vi "Agilent VNA Read Number of Ports.vi"(7 "Agilent VNA":T1, 8 "error in (no error)":errorcluster, 11 "VISA Resource Name":refnum<visa-resource-name>) -> (0 "error out":errorcluster, 2 "Number of Ports":i8, 3 "dup VISA Resource Name":refnum<visa-resource-name>)   [LabVIEW 2011]
doc: "This VI for the HP 8753 is used to read the sweep type.\n\n0 LINEAR FREQ\n1 LOG FREQ\n2 LIST FREQ\n3 CW TIME\n4 POWER SWEEP"
uses:
  TypeDefs/Agilent VNA Instrument Info.ctl
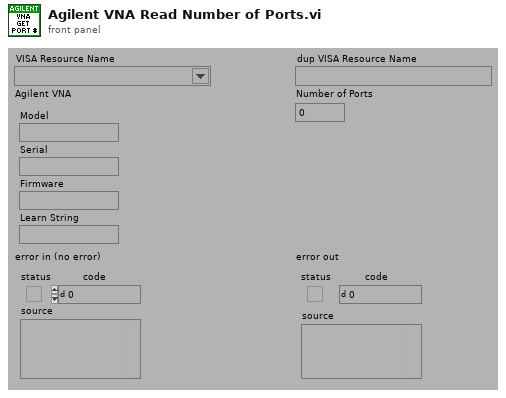
[diagram p1: front panel]
types:
  T1 = typedef "Agilent VNA Instrument Info.ctl" = cluster{"Model":string, "Serial":string, "Firmware":string, "Learn String":string}
  T2 = typedef "Agilent VNA Model.ctl" = enum16{"Not Supported", "8510X", "8719X", "8720X", "8722X", "8753X", "ENA", "PNA", "Field Fox"}
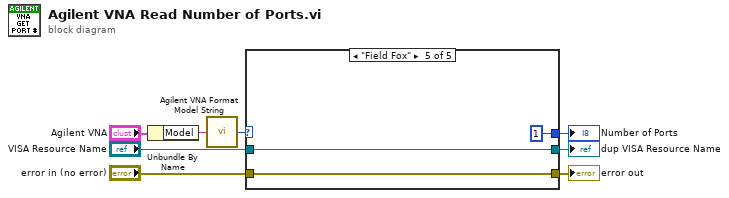
[diagram p0: block diagram]
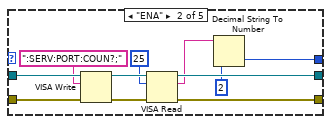
[diagram p3: hidden frame]
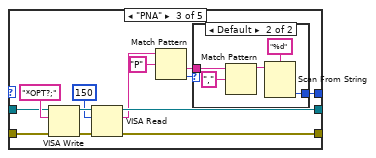
[diagram p4: hidden frame]
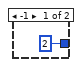
[diagram p5: hidden frame]
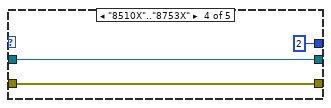
[diagram p6: hidden frame]
diagram:
  n1 = Unbundle By Name("Agilent VNA") -> ("Model"=w1:string)
  n2 = call "Agilent VNA Format Model String.vi"("Model"=w1) -> ("Model"=w3:T2)
  n3 = case shown="\"Field Fox\"" w3 {
    tunnel: "VISA Resource Name" -> [w10 w17 w30 w42 w45]
    tunnel: "error in (no error)" -> [w9 w21 w29 w43 w46]
    tunnel: [w9 w20 w28 w43 w46] -> w7
    tunnel: [_ w12 w23 2 1] -> w6
    tunnel: [w10 w15 w27 w42 w45] -> w4
    frame "Not Supported" {
    }
    frame "ENA" {
      n4 = VISA Write(VISA resource name=w17, write buffer=":SERV:PORT:COUN?;", error in (no error)=w21) -> (VISA resource name out=w18:refnum<visa-resource-name>, error out=w19:errorcluster)  [unwired: 1 out]
      n5 = VISA Read(VISA resource name=w18, byte count=u32 25, error in (no error)=w19) -> (VISA resource name out=w15:refnum<visa-resource-name>, read buffer=w14:string, error out=w20:errorcluster)  [unwired: 1 out]
      n6 = Decimal String To Number(string=w14, default (0L)=i8 2 ("Number of Channels")) -> (number=w12:i8)  [unwired: 2 out]
    }
    frame "PNA" {
      n7 = VISA Write(VISA resource name=w30, write buffer="*OPT?;", error in (no error)=w29) -> (VISA resource name out=w33:refnum<visa-resource-name>, error out=w34:errorcluster)  [unwired: 1 out]
      n8 = VISA Read(VISA resource name=w33, byte count=u32 150, error in (no error)=w34) -> (VISA resource name out=w27:refnum<visa-resource-name>, read buffer=w24:string, error out=w28:errorcluster)  [unwired: 1 out]
      n9 = Match Pattern(string=w24, regular expression="P") -> (after substring=w26:string, offset past match=w22:i32)  [unwired: 3 out]
      n10 = case shown="Default" w22 {
        tunnel: w26 -> [_ w37]
        tunnel: [2 w36] -> w23
        frame -1 {
        }
        frame Default {
          n11 = Match Pattern(string=w37, regular expression=",") -> (before substring=w39:string)  [unwired: 4 out]
          n12 = Scan From String(format string="%d", input string=w39) -> (output 1=w36:i32)  [unwired: 2 in, 4 out]
        }
      }
    }
    frame "8510X".."8753X" {
    }
    frame "Field Fox" {
    }
  }
  "Number of Ports" <- w6
  "dup VISA Resource Name" <- w4
  "error out" <- w7
